vi "Save User Prefs.vi"(8 "error in (no error)":errorcluster, 11 "Historian Charting Manager in":refnum<class "Historian Charting Manager.lvclass">) -> (0 "error out":errorcluster, 3 "Historian Charting Manager out":refnum<class "Historian Charting Manager.lvclass">)   [LabVIEW 2020, in "VolatusGUI.lvlib" / "Historian Charting Manager.lvclass"]
uses:
  Historian Charting Manager.lvclass
  Historian Charting Manager.lvclass/Historian Charting Manager.ctl
  lv-userprefs/User Prefs/PrefsDB/PrefsDB.lvclass
  lv-userprefs/User Prefs/Pref Group/Pref Group.lvclass
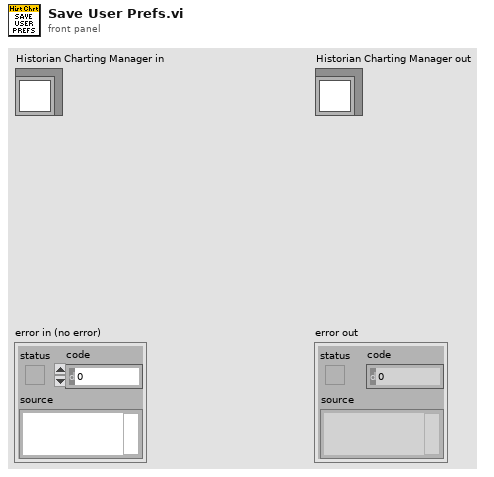
[diagram p1: front panel]
types:
  T1 = typedef "VolatusGUI.lvlib/Historian Charting Manager.lvclass/Plot Group Config.ctl" = cluster{"Name":string, "X-Axis Type":T2, "X-Axis Channel":string, "Plots":T3[], "Lock Now":bool, "Time":string, "Swap Axes":bool}
  T2 = typedef "VolatusGUI.lvlib/Historian Charting Manager.lvclass/X-Axis Type.ctl" = enum16{"Time", "Channel"}
  T3 = typedef "VolatusGUI.lvlib/Historian Charting Manager.lvclass/Plot Config.ctl" = cluster{"Channel":string, "Visible":bool, "Color":u32, "Scale":T4}
  T4 = typedef "VolatusGUI.lvlib/Historian Charting Manager.lvclass/Scale.ctl" = enum16{"Left", "Right"}
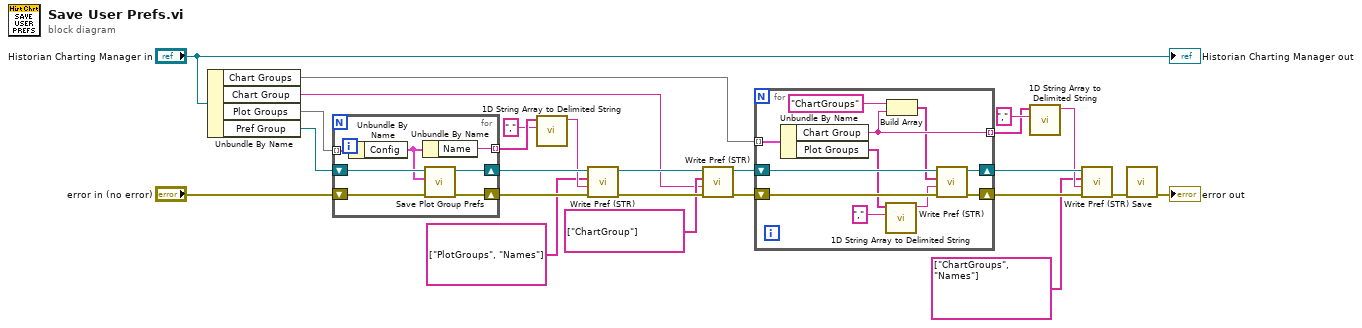
[diagram p0: block diagram]
diagram:
  n1 = Unbundle By Name("Historian Charting Manager in") -> ("Chart Groups"=w9:map{string, string[]}, "Chart Group"=w12:string, "Plot Groups"=w23:map{string, T1}, "Pref Group"=w24:refnum<class "Pref Group.lvclass">)
  n2 = for {
    tunnel: w23 -> [w32] mode=indexing
    shift-right: [w27] -> w21
    shift-left: w24 -> [w31]
    shift-right: [w26] -> w20
    shift-left: "error in (no error)" -> [w30]
    tunnel: [w28] -> w19 mode=indexing
    n3 = Unbundle By Name(w32) -> ("Config"=w29:T1)
    n4 = Unbundle By Name(w29) -> ("Name"=w28:string)
    n5 = call "Save Plot Group Prefs.vi"("error in (no error)"=w30, "Plot Group Config"=w29, "Pref Group in"=w31) -> ("error out"=w26:errorcluster, "Pref Group out"=w27:refnum<class "Pref Group.lvclass">)  [unwired: 7 in]
  }
  n6 = call <vilib>:"1D String Array to Delimited String.vi"("delimiter"=",", "string array"=w19) -> ("delimited string"=w17:string)  [unwired: 9 in]
  n7 = call "Write Pref (STR).vi"("error in (no error)"=w20, "Value"=w17, "Pref Hierarchy"=string[] ["PlotGroups", "Names"], "Pref Group in"=w21) -> ("error out"=w14:errorcluster, "Pref Group out"=w15:refnum<class "Pref Group.lvclass">)  [unwired: 6 in]
  n8 = call "Write Pref (STR).vi"("error in (no error)"=w14, "Value"=w12, "Pref Hierarchy"=string[] ["ChartGroup"], "Pref Group in"=w15) -> ("error out"=w11:errorcluster, "Pref Group out"=w10:refnum<class "Pref Group.lvclass">)  [unwired: 6 in]
  n9 = for {
    shift-right: [w33] -> w7
    shift-left: w11 -> [w43]
    shift-right: [w34] -> w8
    shift-left: w10 -> [w41]
    tunnel: w9 -> [w42] mode=indexing
    tunnel: [w39] -> w3 mode=indexing
    n10 = Unbundle By Name(w42) -> ("Chart Group"=w39:string, "Plot Groups"=w36:string[])
    n11 = call <vilib>:"1D String Array to Delimited String.vi"("delimiter"=",", "string array"=w36) -> ("delimited string"=w35:string)  [unwired: 9 in]
    n12 = Build Array("ChartGroups" ("String"), w39) -> (w38:string[])
    n13 = call "Write Pref (STR).vi"("error in (no error)"=w43, "Value"=w35, "Pref Hierarchy"=w38, "Pref Group in"=w41) -> ("error out"=w33:errorcluster, "Pref Group out"=w34:refnum<class "Pref Group.lvclass">)  [unwired: 6 in]
  }
  n14 = call <vilib>:"1D String Array to Delimited String.vi"("delimiter"=",", "string array"=w3) -> ("delimited string"=w2:string)  [unwired: 9 in]
  n15 = call "Write Pref (STR).vi"("error in (no error)"=w7, "Value"=w2, "Pref Hierarchy"=string[] ["ChartGroups", "Names"], "Pref Group in"=w8) -> ("error out"=w6:errorcluster)  [unwired: 6 in, 1 out]
  n16 = call "Save.vi"("error in (no error)"=w6) -> ("error out"=→"error out":errorcluster)  [unwired: 9 in, 1 out]
  "Historian Charting Manager out" <- "Historian Charting Manager in"
